vi "Get Fiducial Draw Color.vi"(10 "Fiducial Source":T1(ring)) -> (2 "Grid Line Color":u32)   [LabVIEW 2017]
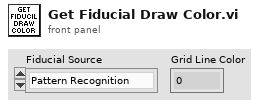
[diagram p1: front panel]
types:
  T1 = enum16{"Pattern Recognition", "User", "Error", "Default"}
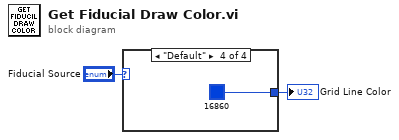
[diagram p0: block diagram]
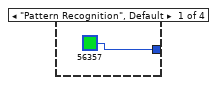
[diagram p2: hidden frame]
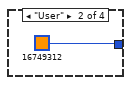
[diagram p3: hidden frame]
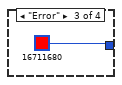
[diagram p4: hidden frame]
diagram:
  n1 = case shown="\"Default\"" "Fiducial Source" {
    tunnel: [u32 56357 ("Grid Line Color") u32 16749312 ("Grid Line Color") u32 16711680 ("Grid Line Color") u32 16860 ("Grid Line Color")] -> w1
    frame "Pattern Recognition", Default {
    }
    frame "User" {
    }
    frame "Error" {
    }
    frame "Default" {
    }
  }
  "Grid Line Color" <- w1
